vi "Nivel de deposito de agua.vi"() -> ()   [LabVIEW 2018]
panel:
  out "data 2":bool[](array[boolean]) caption="data"
  out "data":bool[](array[boolean])
  in  "B":dbl
  in  "A":dbl
  out "Tanque B":dbl(slide) scale=0.0..7.0
  out "Tanque A":dbl(slide) scale=0.0..7.0
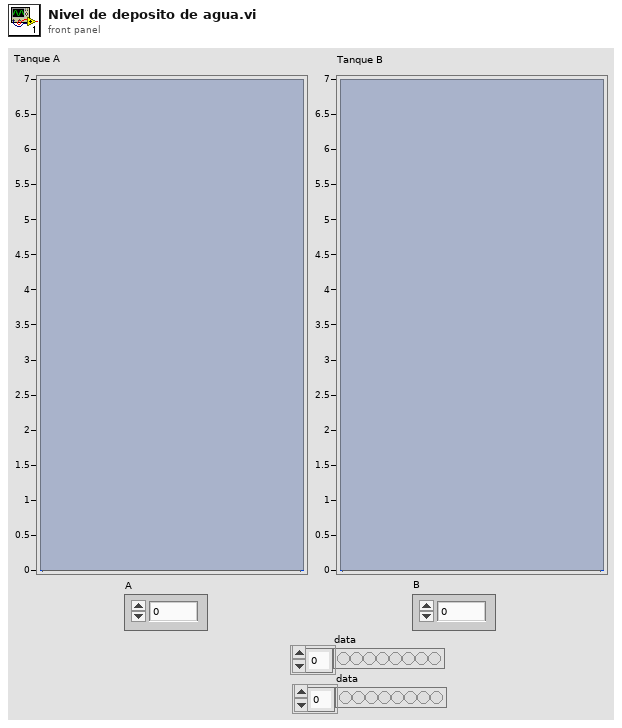
[diagram p1: front panel]
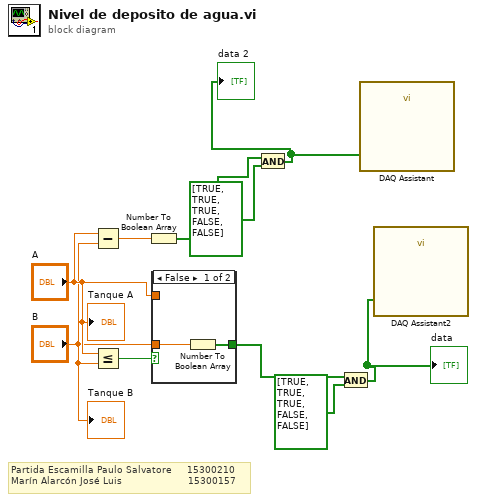
[diagram p0: block diagram]
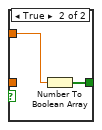
[diagram p2: hidden frame]
diagram:
  # "Partida Escamilla Paulo Salvatore     15300210\nMarín Alarcón José Luis                      15300157"
  n1 = Subtract(x="A", y="B") -> (x-y=w7:dbl)
  n2 = Less Or Equal?(x="A", y="B") -> (x <= y?=w10:bool)
  n3 = Number To Boolean Array(number=w7) -> (Boolean array=w2:bool[])
  n4 = case shown="False" w10 {
    tunnel: "A" -> [_ w14]
    tunnel: [w11 w13] -> w6
    tunnel: "B" -> [w12 _]
    frame False {
      n5 = Number To Boolean Array(number=w12) -> (Boolean array=w11:bool[])
    }
    frame True {
      n6 = Number To Boolean Array(number=w14) -> (Boolean array=w13:bool[])
    }
  }
  n7 = And(x=w2, y=bool[] [TRUE, TRUE, TRUE, FALSE, FALSE]) -> (x .and. y?=w1:bool[])
  "data 2" <- w1
  n8 = And(x=w6, y=bool[] [TRUE, TRUE, TRUE, FALSE, FALSE]) -> (x .and. y?=w4:bool[])
  "data" <- w4
  n9 = call "DAQ Assistant"("data"=w1) -> ()  [unwired: 17 in, 2 out]
  n10 = call "DAQ Assistant2"("data"=w4) -> ()  [unwired: 17 in, 2 out]
  "Tanque A" <- "A"
  "Tanque B" <- "B"
